vi "SRingStartFetch_SD.vi"   [LabVIEW 2015]
uses:
  DLL/ESLSCDLL.dll
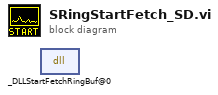
[diagram p0: block diagram]
diagram:
  n1 = dll-call lib="G:/SD/TRANCON-2015/DLL/ESLSCDLL.dll" fn="_DLLStartFetchRingBuf@0" ("lwlscdll.dll:DLLStartFetchRingBuf")() -> ()  [unwired: 4 in, 2 out]
